vi "Main.vi"(11 "Module Admin":refnum<class "Delacor_lib_QMH_Module Admin.lvclass">) -> ()   [LabVIEW 2021, in "Configuration.lvlib"]
doc: "This template is based off of the Queued Message Handler design pattern and the Queued Message Handler project template that ships with LabVIEW.\n\nThe main difference is that the queue is private to this module and communication between modules is performed via Broadcast and Request events.\n\nRequest events are wrapped in public API methods and are handled in the Event Handling Loop (EHL) of this VI. Any module can register for Broadcast events sent by this module. The EHL generates messages based on user interface actions.\n\nThe Message Handling Loop (MHL) processes messages generated by the EHL, or by other messages. The messages are string values, so new messages can be added easily to the Message Cases case structure in the MHL. Each message cluster can also provide an optional value for Message Data, which is a variant that can be converted to whatever message-specific data is required.\n_____\nBased on DQMH Project Template 7.0.1.1316."
uses:
  Configuration.lvlib
  <vilib>/LabVIEW Targets/FPGA/cRIO/shared/nicrio_ModuleControls/nicrio_cRIO-9234_DataRatesRing2.ctl
  <vilib>/LabVIEW Targets/FPGA/cRIO/shared/nicrio_ModuleControls/nicrio_cRIO-9234_ConfigModeRing.ctl
  <vilib>/Delacor/Delacor QMH/Libraries/Module Admin_class/Delacor_lib_QMH_Module Admin.lvclass
  Analog Output/Controls/AO Timing Cluster.ctl
  AI-Current Channel Data's--Cluster.ctl
  AI-Voltage Channel Data's.ctl
  Config-Channel Type.ctl
  Channel Sub-Type.ctl
  AI-Thermocouple Data's.ctl
  Module Data--cluster.ctl
  Host-Control's/Configuration UI Reference.ctl
  DO Channel's.ctl
  <vilib>/Wovalab/Utilities/Helper Loop Periodic Timing/Helper Loop Periodic Timing.lvclass/Helper Loop Periodic Timing.ctl
  Host-Control's/Module ID Action Enum.ctl
  <vilib>/Delacor/Delacor QMH/Libraries/Message Queue_class/Delacor_lib_QMH_Message Queue.lvclass/Delacor_lib_QMH_Message Queue.ctl
  Host-Control's/DTT Test folder Name's.ctl
  Stop Argument--cluster.ctl
  <vilib>/Delacor/Delacor QMH/Libraries/Module Admin_class/Delacor_lib_QMH_Module Admin.lvclass/Delacor_lib_QMH_Module Admin.ctl
  <vilib>/Utility/miscctls.llb/LVPointTypeDef.ctl
  All Interface Data.ctl
  Analog Input Single Channel Data--Cluster.ctl
  Host-Control's/HW Name Enum.ctl
  <vilib>/Delacor/Delacor QMH/Libraries/Message Queue_class/Delacor_lib_QMH_Enqueue Message (Single).vi
  <vilib>/Delacor/Delacor QMH/Libraries/Module Admin_class/Delacor_lib_QMH_Get External Launch.vi
  <vilib>/Wovalab/Utilities/Helper Loop Periodic Timing/U32 Max Value--constant.vi
  <vilib>/Wovalab/Utilities/Helper Loop Periodic Timing/Update Last Execution Time.vi
  <vilib>/Utility/traverseref.llb/TRef Get All FP References.vi
  <vilib>/Utility/traverseref.llb/Get GObject Label.vi
  <vilib>/Utility/xml.llb/Read From XML File.vi
  <vilib>/Utility/xml.llb/Read From XML File(string).vi
  <vilib>/addons/_JKI.lib/Serialization/JSON/Library/Flatten To JSON String.vi
  <vilib>/Wovalab/Utilities/Helper Loop Periodic Timing/Helper Loop Periodic Timing.lvclass
  <vilib>/Delacor/Delacor QMH/Libraries/Message Queue_class/Delacor_lib_QMH_Message Queue.lvclass
  Main-Module/Host Main.lvlib
  RT Acquisition Engine/RT Acquisition Engine.lvlib
  Hardware Selection/Hardware Selection.lvlib
  <userlib>/_OpenG.lib/appcontrol/appcontrol.llb/openg_application_control.lvlib
panel:
  out "element 2":string
  in  "Channel Type's":cluster{"Channel Type":T1, "Sub-Type":T2}
  in  "AI-Acclerometer":T3={"maximum value"=5.0, "minimum value"=-5.0, "input terminal configuration"=-1, "current excitation source"=10200, "current excitation value"=0.004, "units"=10186, "sensitivity"=1000.0, "sensitivity units"=12509} {"sensitivity units" items=["mVolts/g"=12509, "Volts/g"=12510]; "units" items=["g"=10186, "m/s^2"=12470, "in/s^2"=12471, "From Custom Scale"=10065]; "current excitation source" items=["Internal"=10200, "External"=10167, "None"=10230]; "input terminal configuration" items=["default"=-1, "RSE"=10083, "NRSE"=10078, "Differential"=10106, "Pseudodifferential"=12529]; "minimum value" format="%0.2f"; "maximum value" format="%0.2f"}
  in  "Open":bool
  in  "New":bool
  in  "Get Channel List":bool
  in  "Save":bool
  out "Status & Warning's":string
  in  "Refresh":bool
  out "Release":bool
  out "Safety":bool
  out "Capsule-4":bool
  out "Capsule-3":bool
  out "Capsule-2":bool
  out "Array":string[](array[string])
  in  "Chnl Enbl/Dsbl":bool
  in  "Configure":bool
  out "NewVal":string
  in  "Identification Name":string
  out "Capsule-1":bool
  out "sbRIO":bool
  in  "Config":T4(tab)
  in  "AI-Voltage Data's":T5={"input terminal configuration"=-1, "maximum value"=5.0, "minimum value"=-5.0, "units"=10348} {"units" items=["Volts"=10348, "From Custom Scale"=10065]; "minimum value" format="%0.2f"; "maximum value" format="%0.2f"; "input terminal configuration" items=["Default"=-1, "RSE"=10083, "NRSE"=10078, "Differential"=10106, "Pseudodifferential"=12529]}
  in  "Analog Input Timing":T6={"samples per channel"=1000, "sample mode"=10178, "Sampling Rate"=1000.0} {"sample mode" items=["Finite Samples"=10178, "Continuous Samples"=10123, "Hardware Timed Single Point"=12522]}
  in  "AI-Current":T7={"maximum value"=0.01, "minimum value"=-0.01, "input terminal configuration"=-1, "external shunt resistor value"=249.0, "units"=10342, "shunt resistor location"=-1} {"shunt resistor location" items=["default"=-1, "Internal"=10200, "External"=10167]; "units" items=["Amps"=10342, "From Custom Scale"=10065]; "external shunt resistor value" format="%0.2f"; "input terminal configuration" items=["default"=-1, "RSE"=10083, "NRSE"=10078, "Differential"=10106, "Pseudodifferential"=12529]; "minimum value" format="%0.5f"; "maximum value" format="%0.5f"}
  in  "AI-ThermoCouple":T8={"thermocouple type"=10072, "maximum value"=100.0, "minimum value"=0.0, "units"=10143} {"units" items=["Deg C"=10143, "Deg F"=10144, "Kelvins"=10325, "Deg R"=10145, "From Custom Scale"=10065]; "minimum value" format="%0.2f"; "maximum value" format="%0.2f"; "thermocouple type" items=["J"=10072, "K"=10073, "N"=10077, "R"=10082, "S"=10085, "T"=10086, "B"=10047, "E"=10055]}
  in  "Analog Output Timing":T6={"samples per channel"=1000, "sample mode"=10178, "Sampling Rate"=1000.0} {"sample mode" items=["Finite Samples"=10178, "Continuous Samples"=10123, "Hardware Timed Single Point"=12522]}
  out "File Path":path
  in  "Proceed":bool
  in  "Update Button":bool
  in  "Cancel":bool
  in  "Commit":bool
  out "Channel Name":string="PXI-6259/ai0" caption="Identification Name"
  in  "Stop Button":bool
  out "Channel settings":T9(tab)
  in  "9234 Ch1":T10 items=["AC Coupled", "DC Coupled", "IEPE AC Coupled"]
  in  "Calibrate":bool
  out "Amplitude":dbl[][](graph)
  in  "Units 2":string
  in  "Input Range      2":enum16{"+/-10V"}(ring)
  out "Prescaled":dbl format="%0.2f"
  out "Scaled":dbl format="%0.2f"
  in  "Scaling_AI":enum32{"Look up table", "Polynomial"}(tab)
  in  "Lookup table":dbl[][](array[numeric])
  in  "Polynomial":dbl[](array[numeric])
  in  "Input Range":T11(ring)
  in  "Calibrate 2":bool
  in  "Units 3":string
  in  "Analog  Output Diagnostic":dbl caption="Output Value :" format="%#_8g"
  in  "Scaling_AI 2":enum32{"Look up table", "Polynomial"}(tab)
  in  "Lookup table 2":dbl[][](array[numeric])
  in  "Polynomial 2":dbl[](array[numeric])
  in  "Output Range":enum16{"+/-10"}(ring)
  in  "EU Min":dbl=-10.0 format="%#_13g"
  in  "EU Max":dbl=10.0 format="%#_13g"
  out "Digital Diagnostic Input":bool caption="Digital Input"
  in  "Boolean":bool caption="0"
  in  "ThermocoupleType":u16(ring) items=["B", "E", "J", "K", "R", "S", "T", "N"]
  in  "Callender-Van Dusen RTD parameters":cluster{"A":dbl, "B":dbl, "C":dbl, "R0":dbl}
  in  "Units":string
  in  "Temperature":dbl
  in  "rtd tab":enum32{"Look up table", "Polynomial"}(tab)
  in  "rtd lookup":dbl[][](array[numeric])
  in  "rtd poly":dbl[](array[numeric])
  in  "Digital Out":bool caption="0"
  in  "Lead/lag":bool caption="0"
  in  "Parameter":T12
  in  "Sampling Rate_9234":T13=5 items=["51.200 kS/s (NI 9234)"=1, "25.600 kS/s (NI 9234)"=2, "17.067 kS/s (NI 9234)"=3, "12.800 kS/s (NI 9234)"=4, "10.240 kS/s (NI 9234)"=5, "8.533 kS/s (NI 9234)"=6, "7.314 kS/s (NI 9234)"=7, "6.400 kS/s (NI 9234)"=8, "5.689 kS/s (NI 9234)"=9, "5.120 kS/s (NI 9234)"=10, "4.654 kS/s (NI 9234)"=11, "4.267 kS/s (NI 9234)"=12, "3.938 kS/s (NI 9234)"=13, "3.657 kS/s (NI 9234)"=14, "3.413 kS/s (NI 9234)"=15, "3.200 kS/s (NI 9234)"=16, "3.012 kS/s (NI 9234)"=17, "2.845 kS/s (NI 9234)"=18, "2.695 kS/s (NI 9234)"=19, "2.560 kS/s (NI 9234)"=20, "2.438 kS/s (NI 9234)"=21, "2.328 kS/s (NI 9234)"=22, "2.226 kS/s (NI 9234)"=23, "2.133 kS/s (NI 9234)"=24, "2.048 kS/s (NI 9234)"=25, "1.969 kS/s (NI 9234)"=26, "1.896 kS/s (NI 9234)"=27, "1.829 kS/s (NI 9234)"=28, "1.765 kS/s (NI 9234)"=29, "1.707 kS/s (NI 9234)"=30, "1.652 kS/s (NI 9234)"=31]
  in  "Sampling Rate":dbl
  in  "ChannelListTree":string(tree)="PXI1Mod5\\Port0\\Line6" caption="Data Portal: Internal Data"
  out "error out":errorcluster
  out "Status":string
  in  "Simulate MHL Error":bool
  in  "Simulate EHL Error":bool
  # "IIT M Drop Tower Test System"
  # "CHANNEL CONFIGURATION"
  # "If Channel Name"
  # "Analog Input Channel Settings"
  # "Scaling"
  # "Diagnostic panel"
  # "Where prescaled is voltage\n             scaled is EU"
  # "PreScale"
  # "Scaled"
  # "C"
  # "m1"
  # "m2"
  # "m3"
  # "m4"
  # "y=c+(m1)x+(m2)x^2+(m3)x^3+(m4)x^4"
  # "Where y is scaled value(EU)\n             x is  prescaled calue(voltage)"
  # "Analog Output Channel Settings"
  # "Diagnostic panel"
  # "Volts"
  # "Where prescaled is voltage\n             scaled is EU"
  # "Pre scaled"
  # "Scaled"
  # "C"
  # "m1"
  # "m2"
  # "m3"
  # "m4"
  # "y=c+(m1)x+(m2)x^2+(m3)x^3+(m4)x^4"
  # "Where y is scaled value(EU)\n             x is  prescaled Value(voltage)"
  # "Digital Input Channel Settings"
  # "Diagnostic panel"
  # "RTD Channel Settings"
  # "Diagnostic panel"
  # "ON"
  # "OFF"
  # "Temperature Channel Stteings"
  # "Diagnostic panel"
  # "Deg C"
  # "Where prescaled is voltage\n             scaled is EU"
  # "Pre scaled"
  # "Scaled"
  # "C"
  # "m1"
  # "m2"
  # "m3"
  # "m4"
  # "y=c+(m1)x+(m2)x^2+(m3)x^3+(m4)x^4"
  # "Where y is scaled value(EU)\n             x is  prescaled calue(voltage)"
  # "Digital Channel Setting"
  # "Switch"
  # "Lag"
  # "Switch"
  # "Lag"
  # "Hz"
  # "Deg"
  # "Lead"
  # "Lag"
  # "Sampling  Settings"
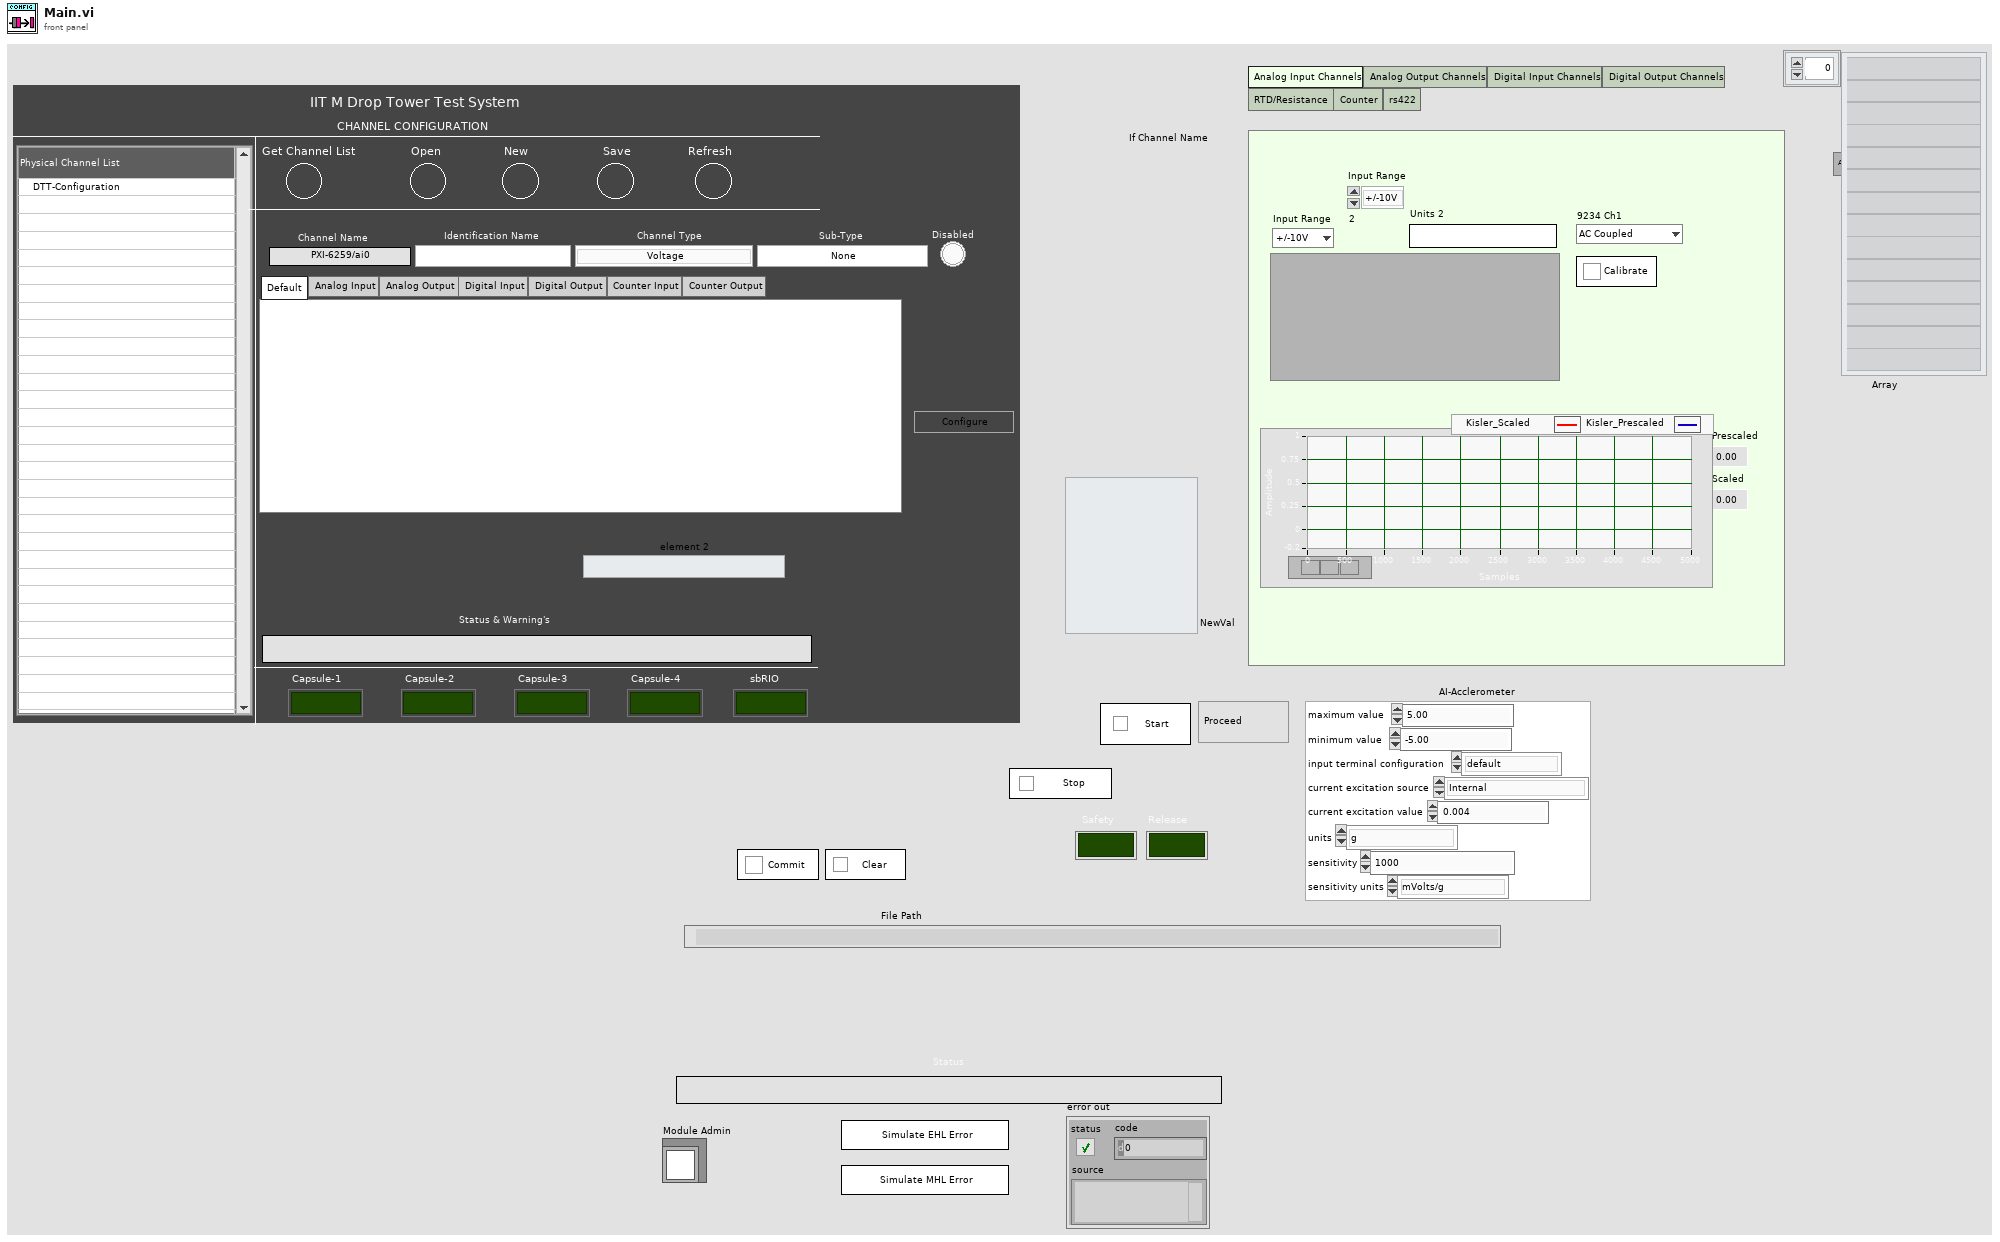
[diagram p1: front panel]
types:
  T1 = typedef "Configuration.lvlib/Config-Channel Type.ctl" = enum16{"Voltage", "Current", "Thermocouple", "Acclerometer"}
  T2 = typedef "Configuration.lvlib/Channel Sub-Type.ctl" = enum16{"None", "Pressure", "Force"}
  T3 = cluster{"maximum value":dbl, "minimum value":dbl, "input terminal configuration":i32, "current excitation source":i32, "current excitation value":dbl, "units":i32, "sensitivity":dbl, "sensitivity units":i32}
  T4 = enum32{"Default", "Analog Input", "Analog Output", "Digital Input", "Digital Output", "Counter Input", "Counter Output"}
  T5 = typedef "Configuration.lvlib/AI-Voltage Channel Data's.ctl" = cluster{"input terminal configuration":i32, "maximum value":dbl, "minimum value":dbl, "units":i32}
  T6 = typedef "AO Timing Cluster.ctl" = cluster{"samples per channel":i32, "sample mode":i32, "Sampling Rate":dbl}
  T7 = typedef "Configuration.lvlib/AI-Current Channel Data's--Cluster.ctl" = cluster{"maximum value":dbl, "minimum value":dbl, "input terminal configuration":i32, "external shunt resistor value":dbl, "units":i32, "shunt resistor location":i32}
  T8 = typedef "Configuration.lvlib/AI-Thermocouple Data's.ctl" = cluster{"thermocouple type":i32, "maximum value":dbl, "minimum value":dbl, "units":i32}
  T9 = enum32{"Analog Input Channels", "Analog Output Channels", "Digital Input Channels", "Digital Output Channels", "RTD/Resistance", "Counter", "rs422"}
  T10 = typedef "nicrio_cRIO-9234_ConfigModeRing.ctl" = u8
  T11 = enum16{"+/-10V", "+/-5V", "+/-2V", "+/-1V", "+/-0.5V", "+/-0.2V", "+/-0.1V"}
  T12 = cluster{"Lead/lag":bool, "Frequency":dbl, "Phase":dbl}
  T13 = typedef "nicrio_cRIO-9234_DataRatesRing2.ctl" = u8
  T14 = typedef "Configuration.lvlib/Request Events--cluster.ctl" = cluster{"Stop Module":refnum<user-event>, "Show Panel":refnum<user-event>, "Hide Panel":refnum<user-event>, "Get Module Execution Status":refnum<user-event>, "Show Diagram":refnum<user-event>}
  T15 = typedef "Configuration.lvlib/Module Data--cluster.ctl" = cluster{"UI Reference":T16, "Tree Selection":cluster{"Selected Channel":string, "Selected Interface":string, "Selected HW":string, "Tree Root Name":string, "Selected Module":string}, "Selected File Path":path, "Selected HW":cluster{"Slctd Hw Name":string[], "Slctd HW IP":string[]}, "Channel Config Path":path, "Interface Data":cluster{"DO Channel's":T17}, "General Info's":cluster{"Idnentification name":string}, "Status":string, "Channel Type's":cluster{"Channel Type":T1, "Sub-Type":T2}, "This VI":refnum<vi>, "Hardware Information ":variant}
  T16 = typedef "Configuration UI Reference.ctl" = cluster{"All Ctrl's Label's":string[], "ChannelListTree":refnum<vi>, "All Object Ref":refnum<vi>[]}
  T17 = typedef "Configuration.lvlib/DO Channel's.ctl" = cluster{"Channel Name":string, "Identification Name":string, "Data":u8[], "Enabled?":bool}[]
  T18 = typedef "Module ID Action Enum.ctl" = enum16{"Init", "Insert", "Get a ID", "Get all ID"}
  T19 = cluster{"Slctd Hw Name":string[], "Slctd HW IP":string[]}
  T20 = typedef "DTT Test folder Name's.ctl" = enum16{"Event Log", "Auto Sequence Configuration", "Channel Configuration's"}
  T21 = enum32{"invalid lock state", "Not Locked", "Locked (No Password)", "Password-protected"}
  T22 = typedef "Configuration.lvlib/Stop Argument--cluster.ctl" = cluster{"Origin":string, "Exit via Stop Module Req?":bool, "Wait for Module to stop?":bool}
  T23 = typedef "LVPointTypeDef.ctl" = cluster{"Horizontal":i16, "Vertical":i16}
  T24 = enum32{"Invalid", "Standard", "Closed", "Hidden", "Minimized", "Maximized"}
  T25 = typedef "HW Name Enum.ctl" = enum16{"Capsule-1", "Capsule-2", "Capsule-3", "Capsule-4", "sb-RIO", "Safety", "Release"}
  T26 = typedef "RT Acquisition Engine.lvlib/Broadcast Events--cluster.ctl" = cluster{"Module Did Init":refnum<user-event>, "Status Updated":refnum<user-event>, "Error Reported":refnum<user-event>, "Module Did Stop":refnum<user-event>, "Update Module Execution Status":refnum<user-event>, "RT Connection Status":refnum<user-event>, "Tx RT Hardware Info":refnum<user-event>, "DO Data's":refnum<user-event>, "AI-Info":refnum<user-event>}
  T27 = typedef "Hardware Selection.lvlib/Broadcast Events--cluster.ctl" = cluster{"Module Did Init":refnum<user-event>, "Status Updated":refnum<user-event>, "Error Reported":refnum<user-event>, "Module Did Stop":refnum<user-event>, "Update Module Execution Status":refnum<user-event>, "Selected RT HW":refnum<user-event>}
  T28 = enum8{"Enabled", "Disabled", "Disabled and Grayed Out"}
  T29 = typedef "Configuration.lvlib/All Interface Data.ctl" = cluster{"DI Config Data":T17, "DO Config Data":T17, "AI Config Data's":cluster{"Module Name":string, "AI Channel's Data":T30[], "Analog Input Timing":T6}[]}
  T30 = typedef "Configuration.lvlib/Analog Input Single Channel Data--Cluster.ctl" = cluster{"Channel Name":string, "Identification Name":string, "Channel Type":T1, "Sub-Type":T2, "Data":string, "Enabled?":bool}
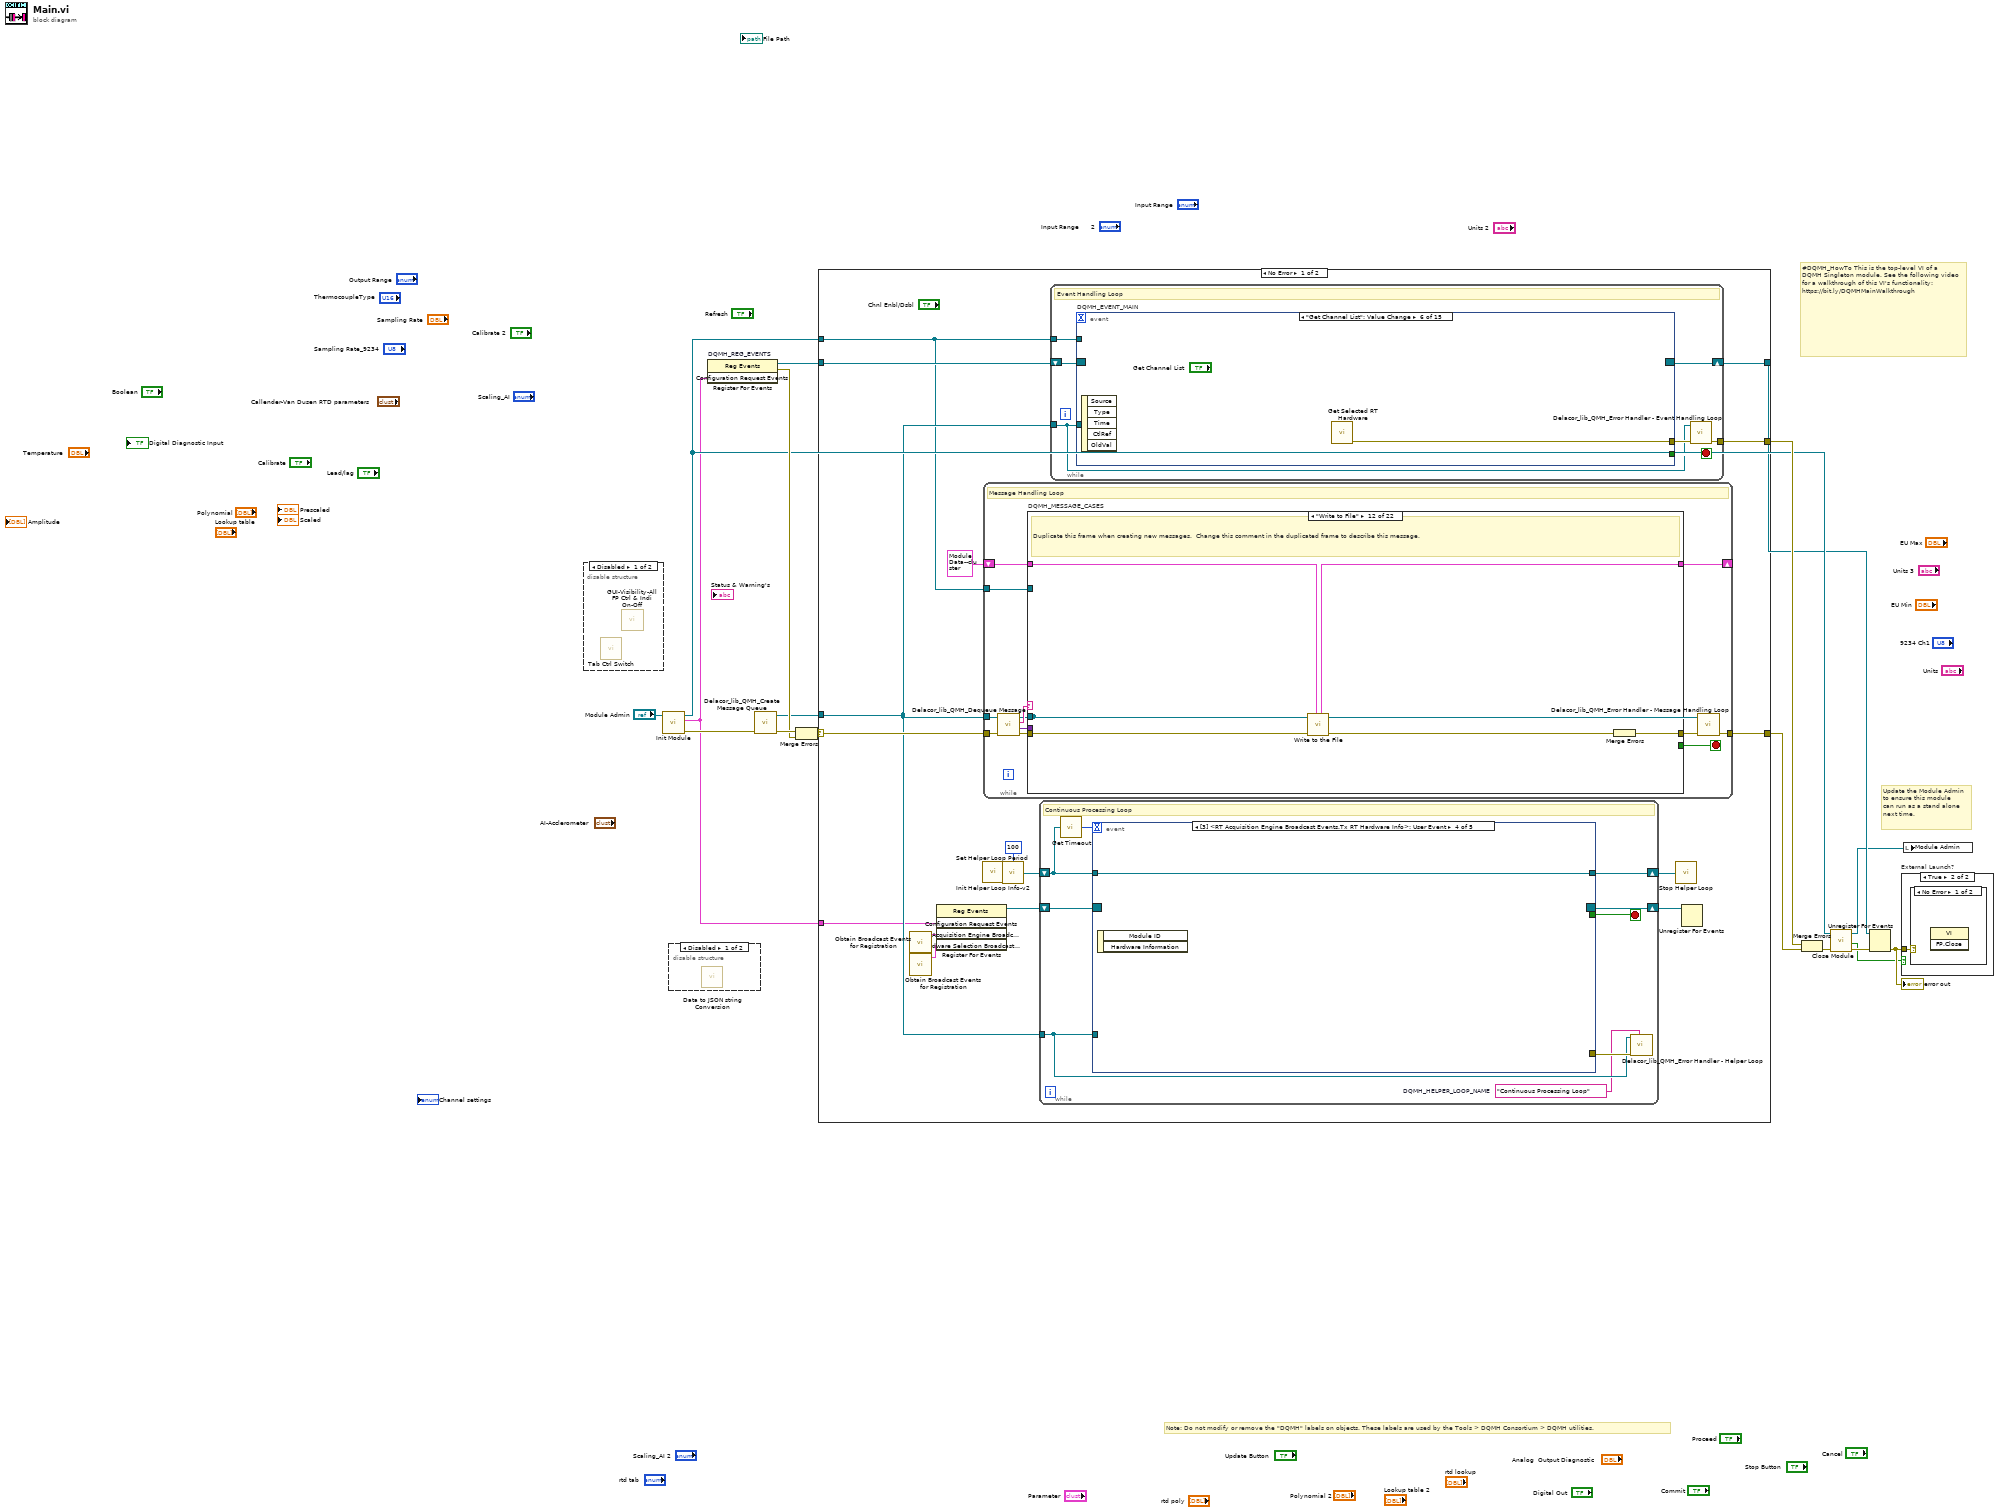
[diagram p0: block diagram]
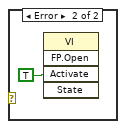
[diagram p5: hidden frame]
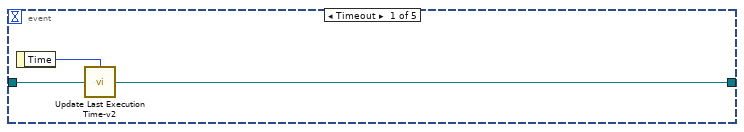
[diagram p6: hidden frame]
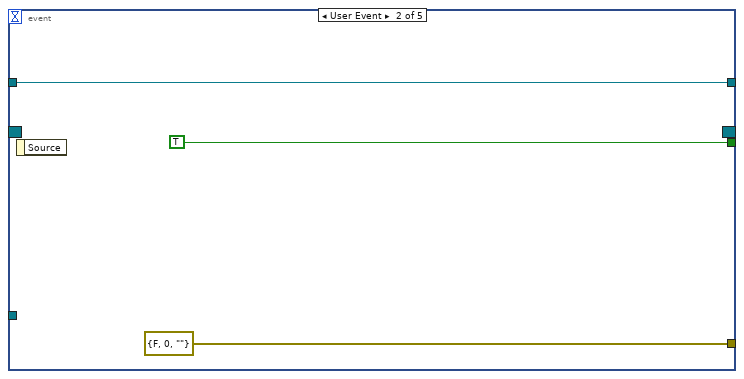
[diagram p7: hidden frame]
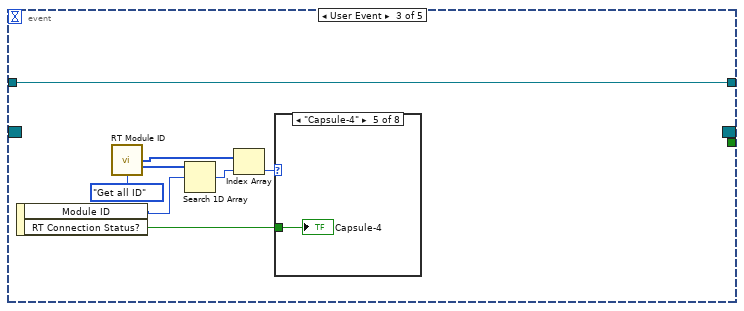
[diagram p8: hidden frame]
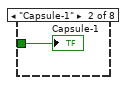
[diagram p10: hidden frame]
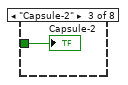
[diagram p11: hidden frame]
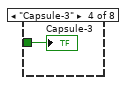
[diagram p12: hidden frame]
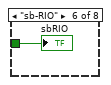
[diagram p13: hidden frame]
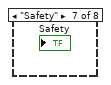
[diagram p14: hidden frame]
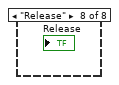
[diagram p15: hidden frame]
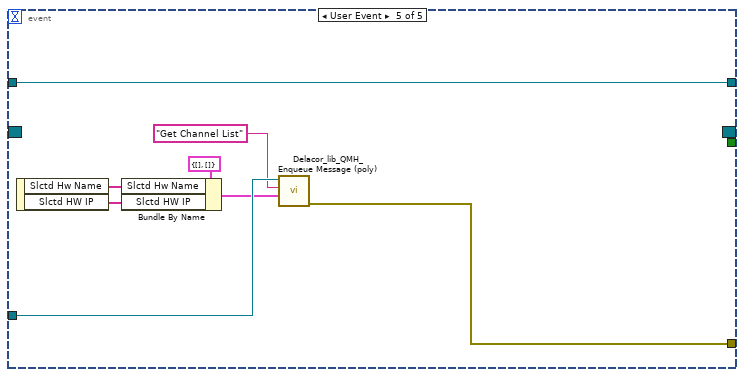
[diagram p16: hidden frame]
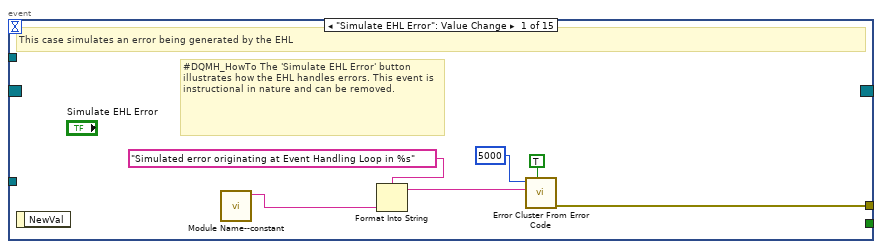
[diagram p17: hidden frame]
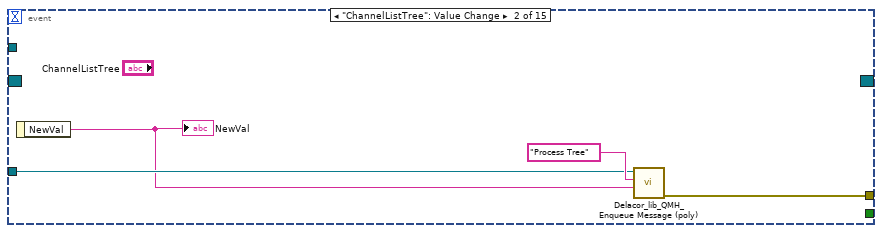
[diagram p18: hidden frame]
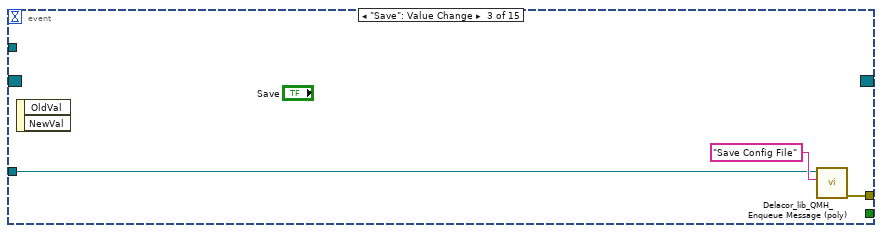
[diagram p19: hidden frame]
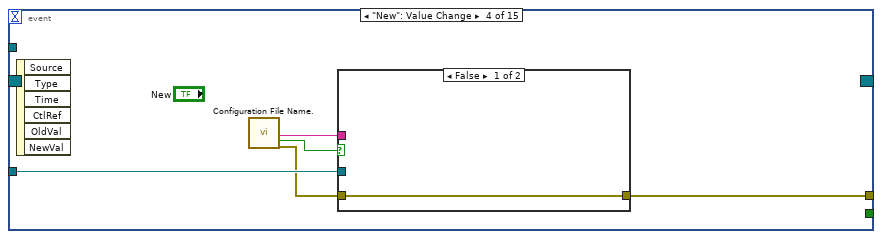
[diagram p20: hidden frame]
diagram:
  # "#DQMH_HowTo This is the top-level VI of a DQMH Singleton module. See the following video for a walkthrough of this VI's functionality: https://bit.ly/DQMHMainWalkthrough"
  # "Note: Do not modify or remove the \"DQMH\" labels on objects. These labels are used by the Tools > DQMH Consortium > DQMH utilities."
  # "Update the Module Admin to ensure this module can run as a stand alone next time."
  n1 = disable-structure shown="Disabled" {
    frame Disabled {
      n2 = call "Tab Ctrl Switch.vi"() -> ()  [unwired: 12 in]
      n3 = call "GUI-Visibility-All FP Ctrl & Indi On-Off.vi"() -> ()  [unwired: 13 in, 3 out]
    }
    frame Enabled {
    }
  }
  n4 = call "Init Module.vi"("Singleton Module Admin in"="Module Admin") -> ("error out"=w16:errorcluster, "Configuration Request Events"=w1:T14, "Singleton Module Admin out"=w8:refnum<class "Delacor_lib_QMH_Module Admin.lvclass">)  [unwired: 8 in]
  n5 = disable-structure shown="Disabled" {
    frame Disabled {
      n6 = call "Data to JSON string Conversion.vi"() -> ()  [unwired: 10 in, 2 out]
    }
    frame Enabled {
    }
  }
  n7 = register-events "DQMH_REG_EVENTS"(w1) -> (reference out=w6:refnum<event-registration>, error out=w9:errorcluster)  [unwired: 2 in]
  n8 = call <vilib>:"Delacor_lib_QMH_Create Message Queue.vi"("error in"=w16) -> ("error out"=w11:errorcluster, "Message Queue"=w5:refnum<class "Delacor_lib_QMH_Message Queue.lvclass">)  [unwired: 9 in]
  n9 = Merge Errors(w11, w9) -> (w10:errorcluster)
  n10 = case shown="No Error" w10 {
    selector: w10 -> [w32 w467]
    tunnel: [w34 w466] -> w17
    tunnel: [w31 w465] -> w7
    tunnel: w6 -> [w29 w465]
    tunnel: w5 -> [w28 w460]
    tunnel: [w33 _] -> w14
    tunnel: w8 -> [w27 w461]
    tunnel: w1 -> [w26 _]
    frame No Error {
      n11 = call "Obtain Broadcast Events for Registration.vi"() -> ("RT Acquisition Engine Broadcast Events"=w19:T26)  [unwired: 9 in, 2 out]
      n12 = call "Obtain Broadcast Events for Registration.vi"() -> ("Hardware Selection Broadcast Events"=w18:T27)  [unwired: 9 in, 2 out]
      n13 = register-events ("DQMH_HELPER_REGFOREVENTS")(w26, w19, w18) -> (reference out=w24:refnum<event-registration>)  [unwired: 2 in, 1 out]
      n14 = call <vilib>:"Init Helper Loop Info-v2.vi"() -> ("Helper Loop Periodic Timing"=w22:refnum<class "Helper Loop Periodic Timing.lvclass">)  [unwired: 1 in]
      n15 = while {
        tunnel: w28 -> [w166]
        shift-right: [w165] -> _
        shift-left: T15 {"UI Reference"={"All Ctrl's Label's"=[], "ChannelListTree"=refnum, "All Object Ref"=[]}, "Tree Selection"={"Selected Channel"="", "Selected Interface"="", "Selected HW"="", "Tree Root Name"="", "Selected Module"=""}, "Selected File Path"=path "", "Selected HW"={"Slctd Hw Name"=[], "Slctd HW IP"=[]}, "Channel Config Path"=path "", "Interface Data"={"DO Channel's"=[]}, "General Info's"={"Idnentification name"=""}, "Status"="", "Channel Type's"={"Channel Type"=enum."Voltage", "Sub-Type"=enum."Pressure"}, "This VI"=refnum, "Hardware Information "=variant(variant[] [])} ("Data Cluster") -> [w174]
        tunnel: w32 -> [w176]
        tunnel: [w169] -> w34
        tunnel: w27 -> [w170]
        stop <- w173 stop-if-true
        # "Message Handling Loop"
        n16 = call-dynamic "Delacor_lib_QMH_Dequeue Message.vi"("error in"=w176, "Message Queue in"=w166) -> ("error out"=w175:errorcluster, "Message Data"=w171:variant, "Message"=w172:string, "Message Queue out"=w167:refnum<class "Delacor_lib_QMH_Message Queue.lvclass">)  [unwired: 6 in]
        n17 = case "DQMH_MESSAGE_CASES" shown="\"Write to File\"" w172 {
          selector: w172 -> [_ _ _ _ _ _ _ _ _ _ _ _ _ _ _ _ _ _ _ _ _ w456]
          tunnel: w167 -> [w187 w210 _ _ _ _ _ w270 _ _ _ _ _ _ w350 _ _ _ _ w422 w443 _]
          tunnel: w175 -> [w203 w208 w246 w255 w258 w261 w264 w283 w302 w306 w320 w326 w333 w337 w347 w401 w406 w408 w417 w428 w449 w458]
          tunnel: [w183 w214 w253 w255 w257 w260 w263 w285 w303 w305 w322 w327 w334 w336 w355 w403 w405 w408 w416 w424 w444 w459] -> w168
          tunnel: w174 -> [w193 w213 w252 w254 w256 w259 w262 w277 w299 w304 w317 w323 w332 w335 w345 w400 w404 w407 w409 w418 w435 w450]
          tunnel: [w181 w206 w250 w254 w256 w259 w262 w273 w300 w304 w316 w324 w329 w335 w342 w398 w404 w407 w409 w418 w435 w450] -> w165
          tunnel: [_ _ _ _ _ _ _ _ _ _ _ _ _ _ _ _ _ _ _ _ w442 _] -> w173
          tunnel: w171 -> [_ _ _ _ _ _ _ w284 _ _ w321 _ _ _ w348 w402 _ _ _ w423 w441 _]
          tunnel: w170 -> [w194 _ _ _ _ _ _ _ _ _ _ _ _ _ _ _ _ _ _ w421 w436 _]
          frame "Initialize" {
            w189 = "Initial Message" ("Initial Message")
            # "Initialize - Any operation that needs to be done before the module can receive messages. Synchronize Caller Events.vi will inform Start Module.vi that the module has launched and is ready to receive messages. Module Did Init.vi will broadcast that the module initialized."
            n18 = call "Synchronize Caller Events.vi"("error in"=w203, "Singleton Module Admin in"=w194) -> ("error out"=w202:errorcluster, "Singleton Module Admin out"=w190:refnum<class "Delacor_lib_QMH_Module Admin.lvclass">)  [unwired: 8 in]
            n19 = property on="Property Node" class="Module Admin"(reference=w190) -> ("Accessors:External Launch"=w198:bool)  [unwired: 1 in, 2 out]
            n20 = Select(t=T24."Hidden" ("State"), s=w198, f=T24."Standard" ("State")) -> (s? t:f=w195:T24)
            n21 = control-ref of="This VI"() -> (w180:refnum<vi>)
            n22 = call "Module Name--constant.vi"() -> ("Module Name"=w201:string)  [unwired: 11 in]
            n23 = property on="Property Node" class="VI"(reference=w180, "Front Panel.Title"=w201) -> (reference out=w200:refnum<vi>, error out=w205:errorcluster)  [unwired: 1 in]
            n24 = call "Module Name--constant.vi"() -> ("Module Name"=w191:string)  [unwired: 11 in]
            n25 = invoke on="Invoke Node" class="VI" method="FP.Open"(reference=w200, error in=w205, "State"=w195) -> (reference out=w199:refnum<vi>, error out=w204:errorcluster)  [unwired: 2 in, 3 out]
            n26 = Bundle By Name(cluster=w193, "Status"=w189, "This VI"=w180) -> (w181:T15)
            n27 = call "Module Did Init.vi"("error in"=w202, "Initialized?"=TRUE, "Origin"=w191) -> ("error out"=w186:errorcluster)  [unwired: 8 in]
            n28 = invoke on="Invoke Node" class="VI" method="FP.Center"(reference=w199, error in=w204) -> (reference out=w178:refnum<vi>, error out=w179:errorcluster)  [unwired: 1 in, 1 out]
            n29 = property on="Pane" class="Pane"("Origin"=T23 {"Horizontal"=0, "Vertical"=0}) -> ()  [unwired: 2 in, 2 out]
            n30 = call <vilib>:"Clear Errors.vi"("error in (no error)"=w179) -> ("error out"=w177:errorcluster)  [unwired: 5 in, 1 out]
            n31 = call <userlib>:"Fit VI window to Largest Dec__ogtk.vi"("error in (no error)"=w177, "VI Ref (calling VI)"=w178) -> ("error out"=w182:errorcluster)  [unwired: 4 in, 1 out]
            n32 = call <vilib>:"Clear Errors.vi"("error in (no error)"=w182) -> ()  [unwired: 5 in, 2 out]
            n33 = call-poly <vilib>:"Delacor_lib_QMH_Enqueue Message (poly).vi"("error in"=w186, "Message"="Init-1", "Message Queue in"=w187) -> ("error out"=w184:errorcluster)  [unwired: 7 in, 1 out]
            n34 = Merge Errors(w184) -> (w183:errorcluster)
            "Status" <- w189
          }
          frame "Init-1" {
            (unwired) T28."Enabled" ("Disabled")
            n35 = for {
              N: 11 -> [_]
              shift-right: [w218] -> w206
              shift-left: w213 -> [w219]
              shift-right: [w216] -> w209
              shift-left: w208 -> [w215]
              i -> [w217]
              n36 = case shown="2" w217 {
                tunnel: w219 -> [w225 w226 w228 w231 w233 w235 w237 w239 w241 w243 w245]
                tunnel: [w224 w226 w228 w231 w233 w235 w237 w239 w241 w243 w245] -> w218
                tunnel: [w220 w227 w229 w230 w232 w234 w236 w238 w240 w242 w244] -> w216
                tunnel: w215 -> [w220 w227 w229 w230 w232 w234 w236 w238 w240 w242 w244]
                frame 0, Default {
                  n37 = control-ref of="Pane"() -> ()  [unwired: 1 out]
                  n38 = control-ref of="ChannelListTree"() -> (w223:refnum<vi>)
                  n39 = call "Folder Creation.vi"("Folder Name"=DTT_Test_folder_Name's."Channel Configuration's") -> ("Selected Folder Path Out"=w221:path)  [unwired: 12 in, 2 out]
                  n40 = Bundle By Name(cluster=w225, "UI Reference.ChannelListTree"=w223, "Channel Config Path"=w221) -> (w224:T15)
                }
                frame 1 {
                  # "General Control's Reference has been bundled in the data cluster"
                }
                frame 2 {
                  # "Analog Input Control's Reference's"
                }
                frame 3 {
                }
                frame 4 {
                }
                frame 5 {
                }
                frame 6 {
                }
                frame 7 {
                }
                frame 8 {
                }
                frame 9 {
                }
                frame 10 {
                }
              }
            }
            n41 = call-poly <vilib>:"Delacor_lib_QMH_Enqueue Message (poly).vi"("error in"=w209, "Message"="Init-2", "Message Queue in"=w210) -> ("error out"=w211:errorcluster)  [unwired: 7 in, 1 out]
            n42 = Merge Errors(w211) -> (w214:errorcluster)
          }
          frame "Init-2" {
            n43 = control-ref of="This VI"() -> (w249:refnum<vi>)
            n44 = call "GUI-Get all FP Ctrl & Indi Label and Ref.vi"("Respected VI Ref"=w249) -> ("All Object Label"=w248:string[], "All Object Ref"=w247:refnum<vi>[])  [unwired: 9 in]
            n45 = Bundle By Name(cluster=w252, "Tree Selection.Tree Root Name"="DTT-Configuration" ("New Root Name"), "UI Reference.All Object Ref"=w247, "UI Reference.All Ctrl's Label's"=w248) -> (w250:T15)
            n46 = Merge Errors(w246) -> (w253:errorcluster)
          }
          frame "---Module Specific---" {
            # "Separator -- The following cases handle messages specific to this Module."
          }
          frame "---Copy This Frame---" {
            # "Duplicate this frame when creating new messages.  Change this comment in the duplicated frame to describe this message."
            n47 = Merge Errors(w258) -> (w257:errorcluster)
          }
          frame "-----General Operation's-----" {
            # "Duplicate this frame when creating new messages.  Change this comment in the duplicated frame to describe this message."
            n48 = Merge Errors(w261) -> (w260:errorcluster)
          }
          frame "-----Tree Operations-----" {
            # "Duplicate this frame when creating new messages.  Change this comment in the duplicated frame to describe this message."
            n49 = Merge Errors(w264) -> (w263:errorcluster)
          }
          frame "Process Tree" {
            # "\\DTT-Configuration\\192.168.32.50\\Analog Input\\Mod3/ai12"
            # "Duplicate this frame when creating new messages.  Change this comment in the duplicated frame to describe this message."
            n50 = Variant To Data(error in=w283, type="", Variant=w284) -> (data=w281:string, error out=w279:errorcluster)
            n51 = Reverse String(1:w281) -> (0:w280:string)
            n52 = while {
              shift-right: [w293] -> _
              shift-left: w280 -> [w298]
              tunnel: [w292] -> w278 mode=indexing
              shift-right: [w291] -> w267
              shift-left: w279 -> [w291]
              stop <- w294 stop-if-true
              n53 = Match Pattern(string=w298, regular expression="\\") -> (before substring=w296:string, after substring=w293:string, offset past match=w295:i32)  [unwired: 1 in, 1 out]
              n54 = Less Than 0?(x=w295) -> (x < 0?=w294:bool)
              n55 = Reverse String(1:w296) -> (0:w292:string)
            }
            "Array" <- w278
            n56 = Index Array(array=w278) -> (element #1=w274:string, element #2=w276:string, element #3=w275:string, element #4=w265:string, element #5=→"element 2":string)  [unwired: 5 in]
            n57 = Bundle By Name(cluster=w277, "Tree Selection.Selected Channel"=w274, "Tree Selection.Selected Module"=w276, "Tree Selection.Selected Interface"=w275, "Tree Selection.Selected HW"=w265) -> (w268:T15)
            n58 = call "Check and Create File.vi"("error in"=w267, "Data Cluster In"=w268) -> ("error out"=w272:errorcluster, "Read File?"=w269:bool, "Data Cluster Out"=w273:T15)  [unwired: 7 in]
            n59 = case shown="False" w269 {
              tunnel: w272 -> [w288 w290]
              tunnel: [w287 w290] -> w271
              tunnel: w270 -> [w286 _]
              frame False {
                n60 = call-poly <vilib>:"Delacor_lib_QMH_Enqueue Message (poly).vi"("error in"=w288, "Message"="Read file & Update GUI", "Message Queue in"=w286) -> ("error out"=w287:errorcluster)  [unwired: 7 in, 1 out]
              }
              frame True {
              }
            }
            n61 = Merge Errors(w271) -> (w285:errorcluster)
          }
          frame "Add HW Info to Tree" {
            # "Duplicate this frame when creating new messages.  Change this comment in the duplicated frame to describe this message."
            n62 = call "Update Tree Data's.vi"("Data Cluster In"=w299, "error in"=w302) -> ("error out"=w301:errorcluster, "Data Cluster Out"=w300:T15)  [unwired: 8 in]
            n63 = Merge Errors(w301) -> (w303:errorcluster)
          }
          frame "-----XML File Operation's-----" {
            # "Duplicate this frame when creating new messages.  Change this comment in the duplicated frame to describe this message."
            n64 = Merge Errors(w306) -> (w305:errorcluster)
          }
          frame "Opened File" {
            w311 = T29 {"DI Config Data"=[], "DO Config Data"=[], "AI Config Data's"=[]} ("Interface Data")
            # "Duplicate this frame when creating new messages.  Change this comment in the duplicated frame to describe this message."
            n65 = Variant To Data(error in=w320, type=path "" ("File Path"), Variant=w321) -> (data=w314:path, error out=w312:errorcluster)
            n66 = call "XML-Read.vi"("error in (no error)"=w312, "Data"=w311, "XML File Path"=w314) -> ("error out"=w308:errorcluster, "Data Out"=w310:variant, "XML File Path(duplicate)"=w313:path)  [unwired: 6 in]
            n67 = Variant To Data(error in=w308, type=w311, Variant=w310) -> (data=w309:T29, error out=w307:errorcluster)
            n68 = call <vilib>:"Get File Extension.vi"("file"=w313) -> ("filename without extension"=w315:string)  [unwired: 6 in, 4 out]
            n69 = call "Write Channel's to Tree.vi"("Data Cluster In"=w317, "error in (no error)"=w307, "Interface Data"=w309, "File Name"=w315) -> ("error out"=w318:errorcluster, "Data Cluster Out"=w316:T15)  [unwired: 6 in]
            n70 = Merge Errors(w318) -> (w322:errorcluster)
          }
          frame "Write to File" {
            # "Duplicate this frame when creating new messages.  Change this comment in the duplicated frame to describe this message."
            n71 = call "Write to the File.vi"("Data Cluster In"=w323, "error in"=w326) -> ("error out"=w325:errorcluster, "Data Cluster Out"=w324:T15)  [unwired: 8 in]
            n72 = Merge Errors(w325) -> (w327:errorcluster)
          }
          frame "Read file & Update GUI" {
            # "Duplicate this frame when creating new messages.  Change this comment in the duplicated frame to describe this message."
            n73 = call "Read File.vi"("error in"=w333, "Data Cluster In"=w332) -> ("error out"=w331:errorcluster, "Data Cluster Out"=w330:T15)  [unwired: 8 in]
            n74 = call "Config-Tab Switch.vi"("error in (no error)"=w331, "Data Cluster In"=w330) -> ("error out"=w328:errorcluster, "Data Cluster Out"=w329:T15)  [unwired: 7 in, 1 out]
            n75 = Merge Errors(w328) -> (w334:errorcluster)
          }
          frame "---Hardware Operation's---" {
            # "Duplicate this frame when creating new messages.  Change this comment in the duplicated frame to describe this message."
            n76 = Merge Errors(w337) -> (w336:errorcluster)
          }
          frame "Get Channel List" {
            w354 = "Hardware" ("Interface")
            # "Duplicate this frame when creating new messages.  Change this comment in the duplicated frame to describe this message."
            n77 = Variant To Data(error in=w347, type=T19 {"Slctd Hw Name"=[], "Slctd HW IP"=[]}, Variant=w348) -> (data=w343:T19, error out=w340:errorcluster)
            n78 = Unbundle By Name(w343) -> ("Slctd Hw Name"=w346:string[])
            n79 = Bundle By Name(cluster=w345, "Selected HW"=w343) -> (w344:T15)
            n80 = call "Data to JSON string Conversion.vi"("error in"=w340, "Command"=w354, "Interface"=w354) -> ("error out"=w339:errorcluster, "Cmd String"=w341:string)  [unwired: 7 in]
            n81 = for {
              tunnel: w346 -> [w359] mode=indexing
              shift-right: [w360] -> w352
              shift-left: w339 -> [w361]
              tunnel: [w358] -> w338 if=w356
              tunnel: w341 -> [w357]
              n82 = case shown="\"Capsule-4\"" w359 {
                tunnel: w361 -> [w363 w370 w377 w384 w391]
                tunnel: [w363 w370 w377 w384 w391] -> w360
                tunnel: [_ w366 w373 w380 w386] -> w358
                tunnel: w357 -> [_ w364 w372 w379 w387]
                tunnel: [FALSE TRUE TRUE TRUE TRUE] -> w356
                frame Default {
                }
                frame "Capsule-1" {
                  n83 = call "RT Module ID.vi"("HW Name"=HW_Name_Enum."Capsule-1", "Action"=Module_ID_Action_Enum."Get a ID") -> ("Module Id Out"=w367:i32)  [unwired: 10 in, 3 out]
                  n84 = call "Hardware Info.vi"("Data In"=w364, "Module ID"=w367) -> ("Hardware Information"=w366:variant)  [unwired: 7 in, 2 out]
                }
                frame "Capsule-2" {
                  n85 = call "RT Module ID.vi"("HW Name"=HW_Name_Enum."Capsule-2", "Action"=Module_ID_Action_Enum."Get a ID") -> ("Module Id Out"=w374:i32)  [unwired: 10 in, 3 out]
                  n86 = call "Hardware Info.vi"("Data In"=w372, "Module ID"=w374) -> ("Hardware Information"=w373:variant)  [unwired: 7 in, 2 out]
                }
                frame "Capsule-3" {
                  n87 = call "RT Module ID.vi"("HW Name"=HW_Name_Enum."Capsule-3", "Action"=Module_ID_Action_Enum."Get a ID") -> ("Module Id Out"=w381:i32)  [unwired: 10 in, 3 out]
                  n88 = call "Hardware Info.vi"("Data In"=w379, "Module ID"=w381) -> ("Hardware Information"=w380:variant)  [unwired: 7 in, 2 out]
                }
                frame "Capsule-4" {
                  n89 = call "RT Module ID.vi"("HW Name"=HW_Name_Enum."Capsule-4", "Action"=Module_ID_Action_Enum."Get a ID") -> ("Module Id Out"=w388:i32)  [unwired: 10 in, 3 out]
                  n90 = call "Hardware Info.vi"("Data In"=w387, "Module ID"=w388) -> ("Hardware Information"=w386:variant)  [unwired: 7 in, 2 out]
                }
              }
            }
            n91 = Bundle By Name(cluster=w344, "Hardware Information"=w338) -> (w342:T15)
            n92 = call-poly <vilib>:"Delacor_lib_QMH_Enqueue Message (poly).vi"("error in"=w352, "Message"="Add HW Info to Tree", "Message Queue in"=w350) -> ("error out"=w351:errorcluster)  [unwired: 7 in, 1 out]
            n93 = Merge Errors(w351) -> (w355:errorcluster)
          }
          frame "Channel Type" {
            # "Duplicate this frame when creating new messages.  Change this comment in the duplicated frame to describe this message."
            n94 = Variant To Data(error in=w401, type=cluster{"Channel Type":T1, "Sub-Type":T2} {"Channel Type"=enum."Voltage", "Sub-Type"=enum."Pressure"} ("Channel Type's"), Variant=w402) -> (data=w396:cluster{"Channel Type":T1, "Sub-Type":T2}, error out=w399:errorcluster)
            n95 = Bundle By Name(cluster=w400, "Channel Type's"=w396) -> (w395:T15)
            n96 = call "Config-Tab Switch.vi"("error in (no error)"=w399, "Data Cluster In"=w395) -> ("error out"=w393:errorcluster, "Config"=w394:T4, "Data Cluster Out"=w398:T15)  [unwired: 7 in]
            n97 = property on="Config" class="TabCtl (strict)"(error in=w393, "Value"=w394) -> (error out=w392:errorcluster)  [unwired: 1 in, 1 out]
            n98 = Merge Errors(w392) -> (w403:errorcluster)
          }
          frame "---File Operation's---" {
            # "Duplicate this frame when creating new messages.  Change this comment in the duplicated frame to describe this message."
            n99 = Merge Errors(w406) -> (w405:errorcluster)
          }
          frame "---Exit and Error Handling---" {
            # "Separator - The following cases handle errors and exit messages."
          }
          frame "Simulate MHL Error" {
            # "#DQMH_HowTo The 'Simulate MHL Error' button  illustrates how the MHL handles errors. This event is instructional in nature and can be removed."
            # "Simulate an error occurring at the MHL"
            n100 = call "Module Name--constant.vi"() -> ("Module Name"=w411:string)  [unwired: 11 in]
            n101 = Format Into String(format string="Simulated error originating at Message Handling Loop in %s", w411) -> (resulting string=w412:string)  [unwired: 2 in, 1 out]
            n102 = call <vilib>:"Error Cluster From Error Code.vi"("show call chain? (False)"=TRUE, "error message (\"\")"=w412, "error code (0)"=5001) -> ("error out"=w415:errorcluster)  [unwired: 6 in]
            n103 = Merge Errors(w417, w415) -> (w416:errorcluster)
          }
          frame "Error" {
            # "#CodeRecommended - If the module is running in standalone mode (External Launch = FALSE), this code will pop up an error dialog and call the 'Exit' message if an error occurs. Add more fine-grained error management here."
            # "Error - Check the error message data and respond accordingly. This message is sent by the \"Error Handler\" VIs at the end of each loop in this application."
            n104 = property on="Property Node" class="Module Admin"(reference=w421) -> ("Accessors:External Launch"=w420:bool)  [unwired: 1 in, 2 out]
            n105 = Variant To Data(error in=w428, type=errorcluster {"status"=FALSE, "code"=0, "source"=""} ("error constant"), Variant=w423) -> (data=w419:errorcluster, error out=w426:errorcluster)
            n106 = local write "error out"(w419) -> ()
            n107 = call "Error Reported.vi"("Error"=w419) -> ()  [unwired: 10 in, 1 out]
            n108 = case shown="False" w420 {
              tunnel: [w433 _] -> w425
              tunnel: w422 -> [w431 _]
              tunnel: w419 -> [w432 _]
              frame False {
                n109 = disable-structure shown="Default" {
                  disable-tunnel: w432 -> [w434 _]
                  frame condition #0 (active) {
                    # "If the module is running standalone, then pop up an error dialog and call the \"Exit\" message."
                    n110 = call <vilib>:"Simple Error Handler.vi"("error in (no error)"=w434) -> ()  [unwired: 4 in, 5 out]
                  }
                  frame condition #1 {
                    # "To prevent the Simple Error Handler VI from being loaded (e.g. when deploying to a Real-Time target), add the Conditional Disable Symbol \"DQMH_Disable_SEH\" to your project and set it to TRUE."
                  }
                }
                n111 = call-poly <vilib>:"Delacor_lib_QMH_Enqueue Message (poly).vi"("Priority Message? (F)"=TRUE, "Message"="Exit", "Message Queue in"=w431) -> ("error out"=w433:errorcluster)  [unwired: 7 in, 1 out]
              }
              frame True {
                # "If the module was launched externally, calling the Error Reported broadcast VI is the only action performed by the \"Error\" message. The module's caller can then process the error appropriately."
              }
            }
            n112 = Merge Errors(w426, w425) -> (w424:errorcluster)
          }
          frame "Exit" {
            w442 = TRUE  # Stop the VI
            # "Release the message queue reference"
            # "Exit - Exit the application."
            n113 = Variant To Data(error in=w449, type=T22 {"Origin"="", "Exit via Stop Module Req?"=FALSE, "Wait for Module to stop?"=FALSE} ("Stop Argument"), Variant=w441) -> (data=w438:T22, error out=w446:errorcluster)
            n114 = control-ref of="This VI"() -> (w437:refnum<vi>)
            n115 = call <vilib>:"Clear Errors.vi"("error in (no error)"=w446, "specific error code to clear (0: all)"=91 ("91: not all Exit messages will have an argument")) -> ("error out"=w448:errorcluster)  [unwired: 4 in, 1 out]
            n116 = call "Handle Exit.vi"("Stop Argument"=w438, "Admin in"=w436, "VI reference"=w437) -> ("error out"=w445:errorcluster)  [unwired: 7 in, 1 out]
            n117 = call-dynamic "Delacor_lib_QMH_Release Message Queue.vi"("error in"=w448, "Message Queue"=w443) -> ("error out"=w447:errorcluster)  [unwired: 9 in]
            n118 = Merge Errors(w447, w445) -> (w444:errorcluster)
            n119 = call "Error Reported.vi"("Error"=w444) -> ()  [unwired: 10 in, 1 out]
          }
          frame Default {
            # "'Default' case only runs if there is a message that isn't defined in any of the other cases.  Output a programming error."
            n120 = call "Module Name--constant.vi"() -> ("Module Name"=w455:string)  [unwired: 11 in]
            n121 = Format Into String(format string="The invalid message string \"%s\" was received in the Message Handling Loop for module \"%s\".", w456, w455) -> (resulting string=w451:string)  [unwired: 2 in, 1 out]
            n122 = call <vilib>:"Error Cluster From Error Code.vi"("show call chain? (False)"=TRUE, "error message (\"\")"=w451, "error code (0)"=1) -> ("error out"=w457:errorcluster)  [unwired: 6 in]
            n123 = Merge Errors(w458, w457) -> (w459:errorcluster)
          }
        }
        n124 = call-dynamic "Delacor_lib_QMH_Error Handler - Message Handling Loop.vi"("error in"=w168, "Message Queue in"=w167) -> ("dup error in"=w169:errorcluster)  [unwired: 8 in, 1 out]
      }
      n125 = call <vilib>:"Set Helper Loop Period.vi"("Period (ms)"=100, "Helper Loop Periodic Timing in"=w22) -> ("Helper Loop Periodic Timing out"=w23:refnum<class "Helper Loop Periodic Timing.lvclass">)  [unwired: 13 in]
      n126 = while "DQMH_HELPER_LOOP" {
        shift-right: [w43] -> w20
        shift-left: w23 -> [w35]
        shift-right: [w41] -> w25
        shift-left: w24 -> [w42]
        tunnel: w28 -> [w38]
        stop <- w40 stop-if-true
        w37 = "Continuous Processing Loop"  # DQMH_HELPER_LOOP_NAME
        # "Continuous Processing Loop"
        n127 = call <vilib>:"Get Timeout.vi"("Helper Loop Periodic Timing"=w35) -> ("Timeout (ms)"=w36:i32)  [unwired: 12 in, 2 out]
        n128 = event "DQMH_HELPER_EVENT_STRUCTURE" shown="[3] <RT Acquisition Engine Broadcast Events.Tx RT Hardware Info>: User Event" {
          selector: w42 -> [_ _ _ _ _]
          dyn-events: [_ _ _ _ _] -> w41
          timeout: w36 -> [_ _ _ _ _]
          tunnel: w35 -> [w45 w49 w57 w63 w71]
          tunnel: [w44 w49 w57 w63 w71] -> w43
          tunnel: [_ TRUE _ _ _] -> w40
          tunnel: [_ errorcluster {"status"=FALSE, "code"=0, "source"=""} ("error constant") _ _ w66] -> w39
          tunnel: w38 -> [_ _ _ _ w67]
          event Timeout {
            n129 = event-data() -> ("Time"=w46:u32)  [unwired: 1 in]
            n130 = call <vilib>:"Update Last Execution Time-v2.vi"("Time"=w46, "Helper Loop Periodic Timing in"=w45) -> ("Helper Loop Periodic Timing out"=w44:refnum<class "Helper Loop Periodic Timing.lvclass">)  [unwired: 12 in, 1 out]
          }
          event User Event {
            n131 = event-data() -> ()  [unwired: 1 in, 1 out]
          }
          event User Event {
            n132 = event-data() -> ("Module ID"=w51:i32, "RT Connection Status?"=w50:bool)  [unwired: 1 in]
            n133 = call "RT Module ID.vi"("Action"=Module_ID_Action_Enum."Get all ID") -> ("All HW Name Out"=w53:T25[], "All HW-ID Out"=w54:i32[])  [unwired: 11 in, 2 out]
            n134 = Search 1D Array(1D array=w54, element=w51) -> (index of element=w55:i32)  [unwired: 1 in]
            n135 = Index Array(array=w53, index=w55) -> (element=w52:T25)
            n136 = case shown="\"Capsule-4\"" w52 {
              tunnel: w50 -> [_ w58 w59 w60 w61 w62 _ _]
              frame Default {
              }
              frame "Capsule-1" {
                "Capsule-1" <- w58
              }
              frame "Capsule-2" {
                "Capsule-2" <- w59
              }
              frame "Capsule-3" {
                "Capsule-3" <- w60
              }
              frame "Capsule-4" {
                "Capsule-4" <- w61
              }
              frame "sb-RIO" {
                "sbRIO" <- w62
              }
              frame "Safety" {
              }
              frame "Release" {
              }
            }
          }
          event User Event {
            n137 = event-data() -> ()  [unwired: 1 in, 2 out]
          }
          event User Event {
            n138 = event-data() -> ("Slctd Hw Name"=w69:string[], "Slctd HW IP"=w68:string[])  [unwired: 1 in]
            n139 = Bundle By Name(cluster=T19 {"Slctd Hw Name"=[], "Slctd HW IP"=[]}, "Slctd Hw Name"=w69, "Slctd HW IP"=w68) -> (w64:T19)
            n140 = call-poly <vilib>:"Delacor_lib_QMH_Enqueue Message (poly).vi"("Message Data"=w64, "Message"="Get Channel List", "Message Queue in"=w67) -> ("error out"=w66:errorcluster)  [unwired: 7 in, 1 out]
          }
        }
        n141 = call-dynamic "Delacor_lib_QMH_Error Handler - Helper Loop.vi"("Error Debug"=w37, "error in"=w39, "Message Queue in"=w38) -> ()  [unwired: 7 in, 2 out]
      }
      n142 = while {
        tunnel: w28 -> [w72]
        shift-right: [w75] -> w31
        shift-left: w29 -> [w76]
        tunnel: [w77] -> w33
        tunnel: w27 -> [w73]
        stop <- w74 stop-if-true
        # "Event Handling Loop"
        n143 = event "DQMH_EVENT_MAIN" shown="[5] \"Get Channel List\": Value Change" {
          selector: w76 -> [_ _ _ _ _ _ _ _ _ _ _ _ _ _ _]
          dyn-events: [_ _ _ _ _ _ _ _ _ _ _ _ _ _ _] -> w75
          timeout: _ -> [_ _ _ _ _ _ _ _ _ _ _ _ _ _ _]
          tunnel: [_ _ _ _ _ _ _ _ _ _ _ _ _ TRUE ("Discard?") _] -> w74
          tunnel: w72 -> [_ w86 w89 w93 w102 _ w114 w117 w119 _ _ _ _ w139 w153]
          tunnel: [w84 w87 w90 w94 w103 w111 w113 w118 w120 _ _ w127 _ w149 w155] -> w78
          tunnel: w73 -> [_ _ _ _ _ _ _ _ _ _ _ _ _ _ w152]
          event "Simulate EHL Error": Value Change {
            # "#DQMH_HowTo The 'Simulate EHL Error' button  illustrates how the EHL handles errors. This event is instructional in nature and can be removed."
            # "This case simulates an error being generated by the EHL"
            n144 = event-data() -> ()  [unwired: 1 in, 1 out]
            n145 = call "Module Name--constant.vi"() -> ("Module Name"=w81:string)  [unwired: 11 in]
            n146 = Format Into String(format string="Simulated error originating at Event Handling Loop in %s", w81) -> (resulting string=w82:string)  [unwired: 2 in, 1 out]
            n147 = call <vilib>:"Error Cluster From Error Code.vi"("show call chain? (False)"=TRUE, "error message (\"\")"=w82, "error code (0)"=5000) -> ("error out"=w84:errorcluster)  [unwired: 6 in]
          }
          event "ChannelListTree": Value Change {
            n148 = event-data() -> ("NewVal"=w85:string)  [unwired: 1 in]
            "NewVal" <- w85
            n149 = call-poly <vilib>:"Delacor_lib_QMH_Enqueue Message (poly).vi"("Message Data"=w85, "Message"="Process Tree", "Message Queue in"=w86) -> ("error out"=w87:errorcluster)  [unwired: 7 in, 1 out]
          }
          event "Save": Value Change {
            n150 = event-data() -> ()  [unwired: 1 in, 2 out]
            n151 = call-poly <vilib>:"Delacor_lib_QMH_Enqueue Message (poly).vi"("Message"="Save Config File", "Message Queue in"=w89) -> ("error out"=w90:errorcluster)  [unwired: 8 in, 1 out]
          }
          event "New": Value Change {
            n152 = event-data() -> ()  [unwired: 1 in, 6 out]
            n153 = call "Configuration File Name."() -> ("File Name"=w95:string, "OK"=w96:bool, "error out"=w92:errorcluster)  [unwired: 17 in]
            n154 = case shown="False" w96 {
              tunnel: w95 -> [_ _]
              tunnel: [w97 _] -> w94
              tunnel: w93 -> [_ _]
              tunnel: w92 -> [w97 _]
              frame False {
              }
              frame True {
              }
            }
          }
          event "Open": Value Change {
            n155 = event-data() -> ()  [unwired: 1 in, 6 out]
            n156 = call "Folder Creation.vi"("Folder Name"=DTT_Test_folder_Name's."Channel Configuration's") -> ("Selected Folder Path Out"=w98:path, "error out"=w99:errorcluster)  [unwired: 12 in, 1 out]
            n157 = call "File Dialog"("start path"=w98, "error in"=w99) -> ("selected path"=w104:path, "cancelled"=w105:bool, "error out"=w101:errorcluster)  [unwired: 10 in, 1 out]
            n158 = case shown="True" w105 {
              tunnel: w104 -> [w106 _]
              tunnel: [w109 _] -> w103
              tunnel: w102 -> [w108 _]
              tunnel: w101 -> [w107 _]
              frame False {
                n159 = call-poly <vilib>:"Delacor_lib_QMH_Enqueue Message (poly).vi"("error in"=w107, "Message Data"=w106, "Message"="Opened File", "Message Queue in"=w108) -> ("error out"=w109:errorcluster)  [unwired: 6 in, 1 out]
              }
              frame True {
                # "User Pressed the Cancel Button so we no need to open any file's or folder."
              }
            }
          }
          event "Get Channel List": Value Change {
            n160 = event-data() -> ()  [unwired: 1 in, 5 out]
            n161 = call "Get Selected RT Hardware.vi"() -> ("error out"=w111:errorcluster)  [unwired: 11 in]
          }
          event "Channel Type's": Value Change {
            n162 = event-data() -> ("NewVal"=w112:cluster{"Channel Type":T1, "Sub-Type":T2})  [unwired: 1 in]
            n163 = call-poly <vilib>:"Delacor_lib_QMH_Enqueue Message (poly).vi"("Message Data"=w112, "Message"="Channel Type", "Message Queue in"=w114) -> ("error out"=w113:errorcluster)  [unwired: 7 in, 1 out]
          }
          event "Simulate MHL Error": Value Change {
            # "#DQMH_HowTo The 'Simulate MHL Error' button  illustrates how the MHL handles errors. This event is instructional in nature and can be removed."
            # "This case simulates an error being generated by the MHL"
            n164 = event-data() -> ()  [unwired: 1 in, 1 out]
            n165 = call-poly <vilib>:"Delacor_lib_QMH_Enqueue Message (poly).vi"("Message"="Simulate MHL Error", "Message Queue in"=w117) -> ("error out"=w118:errorcluster)  [unwired: 8 in, 1 out]
          }
          event "Configure": Value Change {
            n166 = event-data() -> ()  [unwired: 1 in, 1 out]
            n167 = call-poly <vilib>:"Delacor_lib_QMH_Enqueue Message (poly).vi"("Message"="Write to File", "Message Queue in"=w119) -> ("error out"=w120:errorcluster)  [unwired: 8 in, 1 out]
          }
          event User Event {
            # "Show the panel of this VI, and send a status updated message to let listeners know."
            # "Another Module called the \"Show Panel\" API Method."
            n168 = event-data() -> ()  [unwired: 1 in, 1 out]
            n169 = control-ref of="This VI"() -> (w123:refnum<vi>)
            n170 = call "Open VI Panel.vi"("VI"=w123) -> ()  [unwired: 10 in, 1 out]
            n171 = call "Status Updated.vi"("Status"="Panel shown." ("format string")) -> ()  [unwired: 10 in, 1 out]
          }
          event User Event {
            # "Hide the panel of this VI, and send a status updated message to let listeners know."
            # "Another Module called the \"Hide Panel\" API Method."
            n172 = event-data() -> ()  [unwired: 1 in, 1 out]
            n173 = control-ref of="This VI"() -> (w125:refnum<vi>)
            n174 = call "Hide VI Panel.vi"("VI"=w125) -> ()  [unwired: 10 in, 1 out]
            n175 = call "Status Updated.vi"("Status"="Panel hidden." ("format string")) -> ()  [unwired: 10 in, 1 out]
          }
          event User Event {
            # "Another Module called the \"Get Module Execution Status\" API Method."
            n176 = event-data() -> ()  [unwired: 1 in, 1 out]
            n177 = call "Update Module Execution Status.vi"("Running?"=TRUE) -> ("error out"=w127:errorcluster)  [unwired: 10 in]
          }
          event User Event {
            # "Another Module called the \"Show Diagram\" API Method. This event is used for debugging."
            n178 = event-data() -> ()  [unwired: 1 in, 1 out]
            n179 = disable-structure shown="RUN_TIME_ENGINE==False" {
              frame condition #0 (active) {
                # "functionality not available in exe"
                n180 = invoke on="Invoke Node" class="VI" method="Lock State.Get"() -> (error out=w133:errorcluster, "Get Lock State"=w132:T21, "pwd in cache"=w129:bool)  [unwired: 4 in, 1 out]
                n181 = Equal?(x=T21."Password-protected", y=w132) -> (x = y?=w130:bool)
                n182 = Compound Arithmetic op=AND(w130, invert w129) -> (w128:bool)
                n183 = case shown="False" w128 {
                  tunnel: w133 -> [w136 _]
                  frame False {
                    n184 = property on="Property Node" class="VI"(error in=w136, "BDWin.Open"=TRUE ("Block Diagram Window:Open")) -> ()  [unwired: 1 in, 2 out]
                    n185 = call "Status Updated.vi"("Status"="Block Diagram shown." ("format string")) -> ()  [unwired: 10 in, 1 out]
                  }
                  frame True {
                    # "Password-protected VI, and the password is not in the cache. Do not show the diagram."
                  }
                }
              }
              frame condition #1 {
              }
            }
          }
          event User Event {
            # "The Stop Module Event can get fired from the Exit message in the MHL. The queue gets destroyed in that case. If the queue no longer exists, the Enqueue Exit as a priority message will return error 1. It is safe to ignore, because the module is already exiting."
            # "Another Module called the \"Stop Module\" API Method  or the Message Handling Loop below."
            n186 = event-data() -> ("Origin"=w146:string, "Exit via Stop Module Req?"=w142:bool, "Wait for Module to stop?"=w141:bool)  [unwired: 1 in]
            n187 = Bundle By Name(cluster=T22 {"Origin"="", "Exit via Stop Module Req?"=FALSE, "Wait for Module to stop?"=FALSE} ("Stop Argument"), "Exit via Stop Module Req?"=w142, "Wait for Module to stop?"=w141) -> (w140:T22)
            n188 = local write "Status"(w146) -> ()
            n189 = call-dynamic "Delacor_lib_QMH_Flush Messages.vi"("Message Queue in"=w139) -> ("error out"=w137:errorcluster, "Message Queue out"=w138:refnum<class "Delacor_lib_QMH_Message Queue.lvclass">)  [unwired: 7 in, 2 out]
            n190 = call-poly <vilib>:"Delacor_lib_QMH_Enqueue Message (poly).vi"("Priority Message? (F)"=TRUE, "error in"=w137, "Message Data"=w140, "Message"="Exit", "Message Queue in"=w138) -> ("error out"=w150:errorcluster)  [unwired: 5 in, 1 out]
            n191 = call <vilib>:"Clear Errors.vi"("error in (no error)"=w150, "specific error code to clear (0: all)"=1) -> ("error out"=w149:errorcluster)  [unwired: 4 in, 1 out]
          }
          event Panel Close? {
            w154 = TRUE  # Discard the event, the MHL is responsible for closing and stopping this VI.
            # "Hide the panel or send the 'Exit' message if the user clicks the 'X' on the module main VI panel."
            n192 = event-data() -> ()  [unwired: 1 in, 1 out]
            n193 = property on="Property Node" class="Module Admin"(reference=w152) -> ("Accessors:External Launch"=w151:bool)  [unwired: 1 in, 2 out]
            n194 = case shown="True" w151 {
              tunnel: w153 -> [_ w163]
              tunnel: [w156 w164] -> w155
              frame True {
                # "If externally launched, clicking the 'X' hides the panel, but doesn't close it."
                n195 = control-ref of="This VI"() -> (w160:refnum<vi>)
                n196 = call "Hide VI Panel.vi"("VI"=w160) -> ("error out"=w158:errorcluster)  [unwired: 10 in]
                n197 = call "Status Updated.vi"("error in"=w158, "Status"="Panel hidden." ("format string")) -> ("error out"=w157:errorcluster)  [unwired: 9 in]
                n198 = call "Show Panel.vi"("error in"=w157) -> ("error out"=w156:errorcluster)  [unwired: 10 in]
              }
              frame False {
                # "If run as a stand-alone VI, clicking the panel 'X' stops the VI."
                n199 = call-poly <vilib>:"Delacor_lib_QMH_Enqueue Message (poly).vi"("Priority Message? (F)"=TRUE, "Message"="Exit", "Message Queue in"=w163) -> ("error out"=w164:errorcluster)  [unwired: 7 in, 1 out]
              }
            }
            n200 = event-data ("Event Filter Node")("Discard?"=w154) -> ()  [unwired: 1 in, 1 out]
          }
        }
        n201 = call-dynamic "Delacor_lib_QMH_Error Handler - Event Handling Loop.vi"("error in"=w78, "Message Queue in"=w72) -> ("dup error in"=w77:errorcluster)  [unwired: 8 in, 1 out]
      }
      n202 = call <vilib>:"Stop Helper Loop.vi"("Helper Loop Periodic Timing in"=w20) -> ()  [unwired: 1 out]
      n203 = Unregister For Events(event registration refnum=w25) -> ()  [unwired: 1 in, 1 out]
    }
    frame Error {
      # "Synchronize Caller Events.vi will inform Start Module.vi that the module has launched and will let the code calling Start Module.vi register for broadcasts and would permit the caller receive the broadcast that an error occurred at launch time."
      n204 = call-dynamic "Delacor_lib_QMH_Release Message Queue.vi"("error in"=w467, "Message Queue"=w460) -> ("error out"=w466:errorcluster)  [unwired: 9 in]
      n205 = call "Synchronize Caller Events.vi"("Singleton Module Admin in"=w461) -> ("error out"=w468:errorcluster)  [unwired: 9 in, 1 out]
      n206 = call "Module Name--constant.vi"() -> ("Module Name"=w464:string)  [unwired: 11 in]
      n207 = Format Into String(format string="An error occurred during initialization. %s is no longer running.", w464) -> (resulting string=w462:string)  [unwired: 2 in, 1 out]
      n208 = Merge Errors(w466, w468) -> (w469:errorcluster)
      n209 = call "Error Reported.vi"("Additional Information"=w462, "Error"=w469) -> ()  [unwired: 9 in, 1 out]
    }
  }
  n210 = Merge Errors(w14, w17) -> (w13:errorcluster)
  n211 = call "Close Module.vi"("error in"=w13, "Module Admin in"=w8) -> ("error out"=w15:errorcluster, "External Launch"=w2:bool, "Module Admin out"=w3:refnum<class "Delacor_lib_QMH_Module Admin.lvclass">)  [unwired: 7 in]
  n212 = Unregister For Events(event registration refnum=w7, error in=w15) -> (error out=w12:errorcluster)
  "error out" <- w12
  n213 = case "External Launch?" shown="True" w2 {
    tunnel: w12 -> [_ w470]
    frame False {
    }
    frame True {
      n214 = case shown="No Error" w470 {
        frame No Error {
          n215 = invoke on="Invoke Node" class="VI" method="FP.Close"() -> ()  [unwired: 3 in, 3 out]
        }
        frame Error {
          n216 = invoke on="Invoke Node" class="VI" method="FP.Open"("Activate"=TRUE ("Activate?")) -> ()  [unwired: 4 in, 5 out]
        }
      }
    }
  }
  n217 = local write "Module Admin"(w3) -> ()
